vi "Teleop.vi"(10 "Match Info":T1={"Autonomous Elapsed Seconds"=0.0, "TeleOp Elapsed Seconds"=0.0, "Disabled Elapsed Seconds"=0.0, "Visited Autonomous"=FALSE, "Visited TeleOp"=FALSE, "Visited Disabled"=FALSE, "Autonomous Settings"={"Autonomous Style"=enum."Independent", "VI Refnum"=refnum}}, 11 "Call Context":T2) -> ()   [LabVIEW 2017]
doc: "This VI is called for each enabled TeleOp packet received from the DS. It is typically used to read from joysticks and other inputs and update I/O or setpoints for timed control loops. It should complete and return within 20 milliseconds or risk missing DS packets."
uses:
  <vilib>/Rock Robotics/WPI/DriverStation/WPI_DriverStationDerivedRobotMode.ctl
  <vilib>/Rock Robotics/WPI/DriverStation/WPI_DriverStationMatch Info.ctl
  <vilib>/Rock Robotics/WPI/Utilities/WPI_GetSetVariantRefNum.vi
  <vilib>/Rock Robotics/Network Tables/NT Write Boolean Array.vi
  <vilib>/Rock Robotics/Network Tables/NT Write Numeric Array.vi
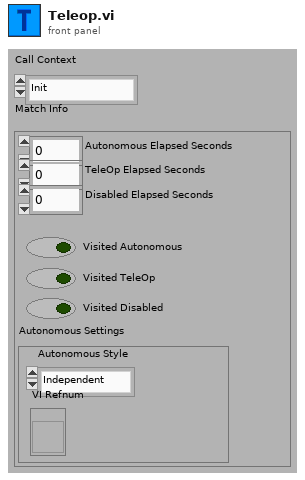
[diagram p1: front panel]
types:
  T1 = typedef "WPI_DriverStationMatch Info.ctl" = cluster{"Autonomous Elapsed Seconds":dbl, "TeleOp Elapsed Seconds":dbl, "Disabled Elapsed Seconds":dbl, "Visited Autonomous":bool, "Visited TeleOp":bool, "Visited Disabled":bool, "Autonomous Settings":cluster{"Autonomous Style":enum16{"Iterative", "Independent"}, "VI Refnum":refnum<vi>}}
  T2 = typedef "WPI_DriverStationDerivedRobotMode.ctl" = enum16{"Init", "Execute", "Stop"}
  T3 = typedef "WPI_JoystickDevRef.ctl" = cluster{"Device":T4}
  T4 = typedef "WPI_JoystickDeviceEnum.ctl" = enum16{"USB 0", "USB 1", "USB 2", "USB 3", "USB 4", "USB 5"}
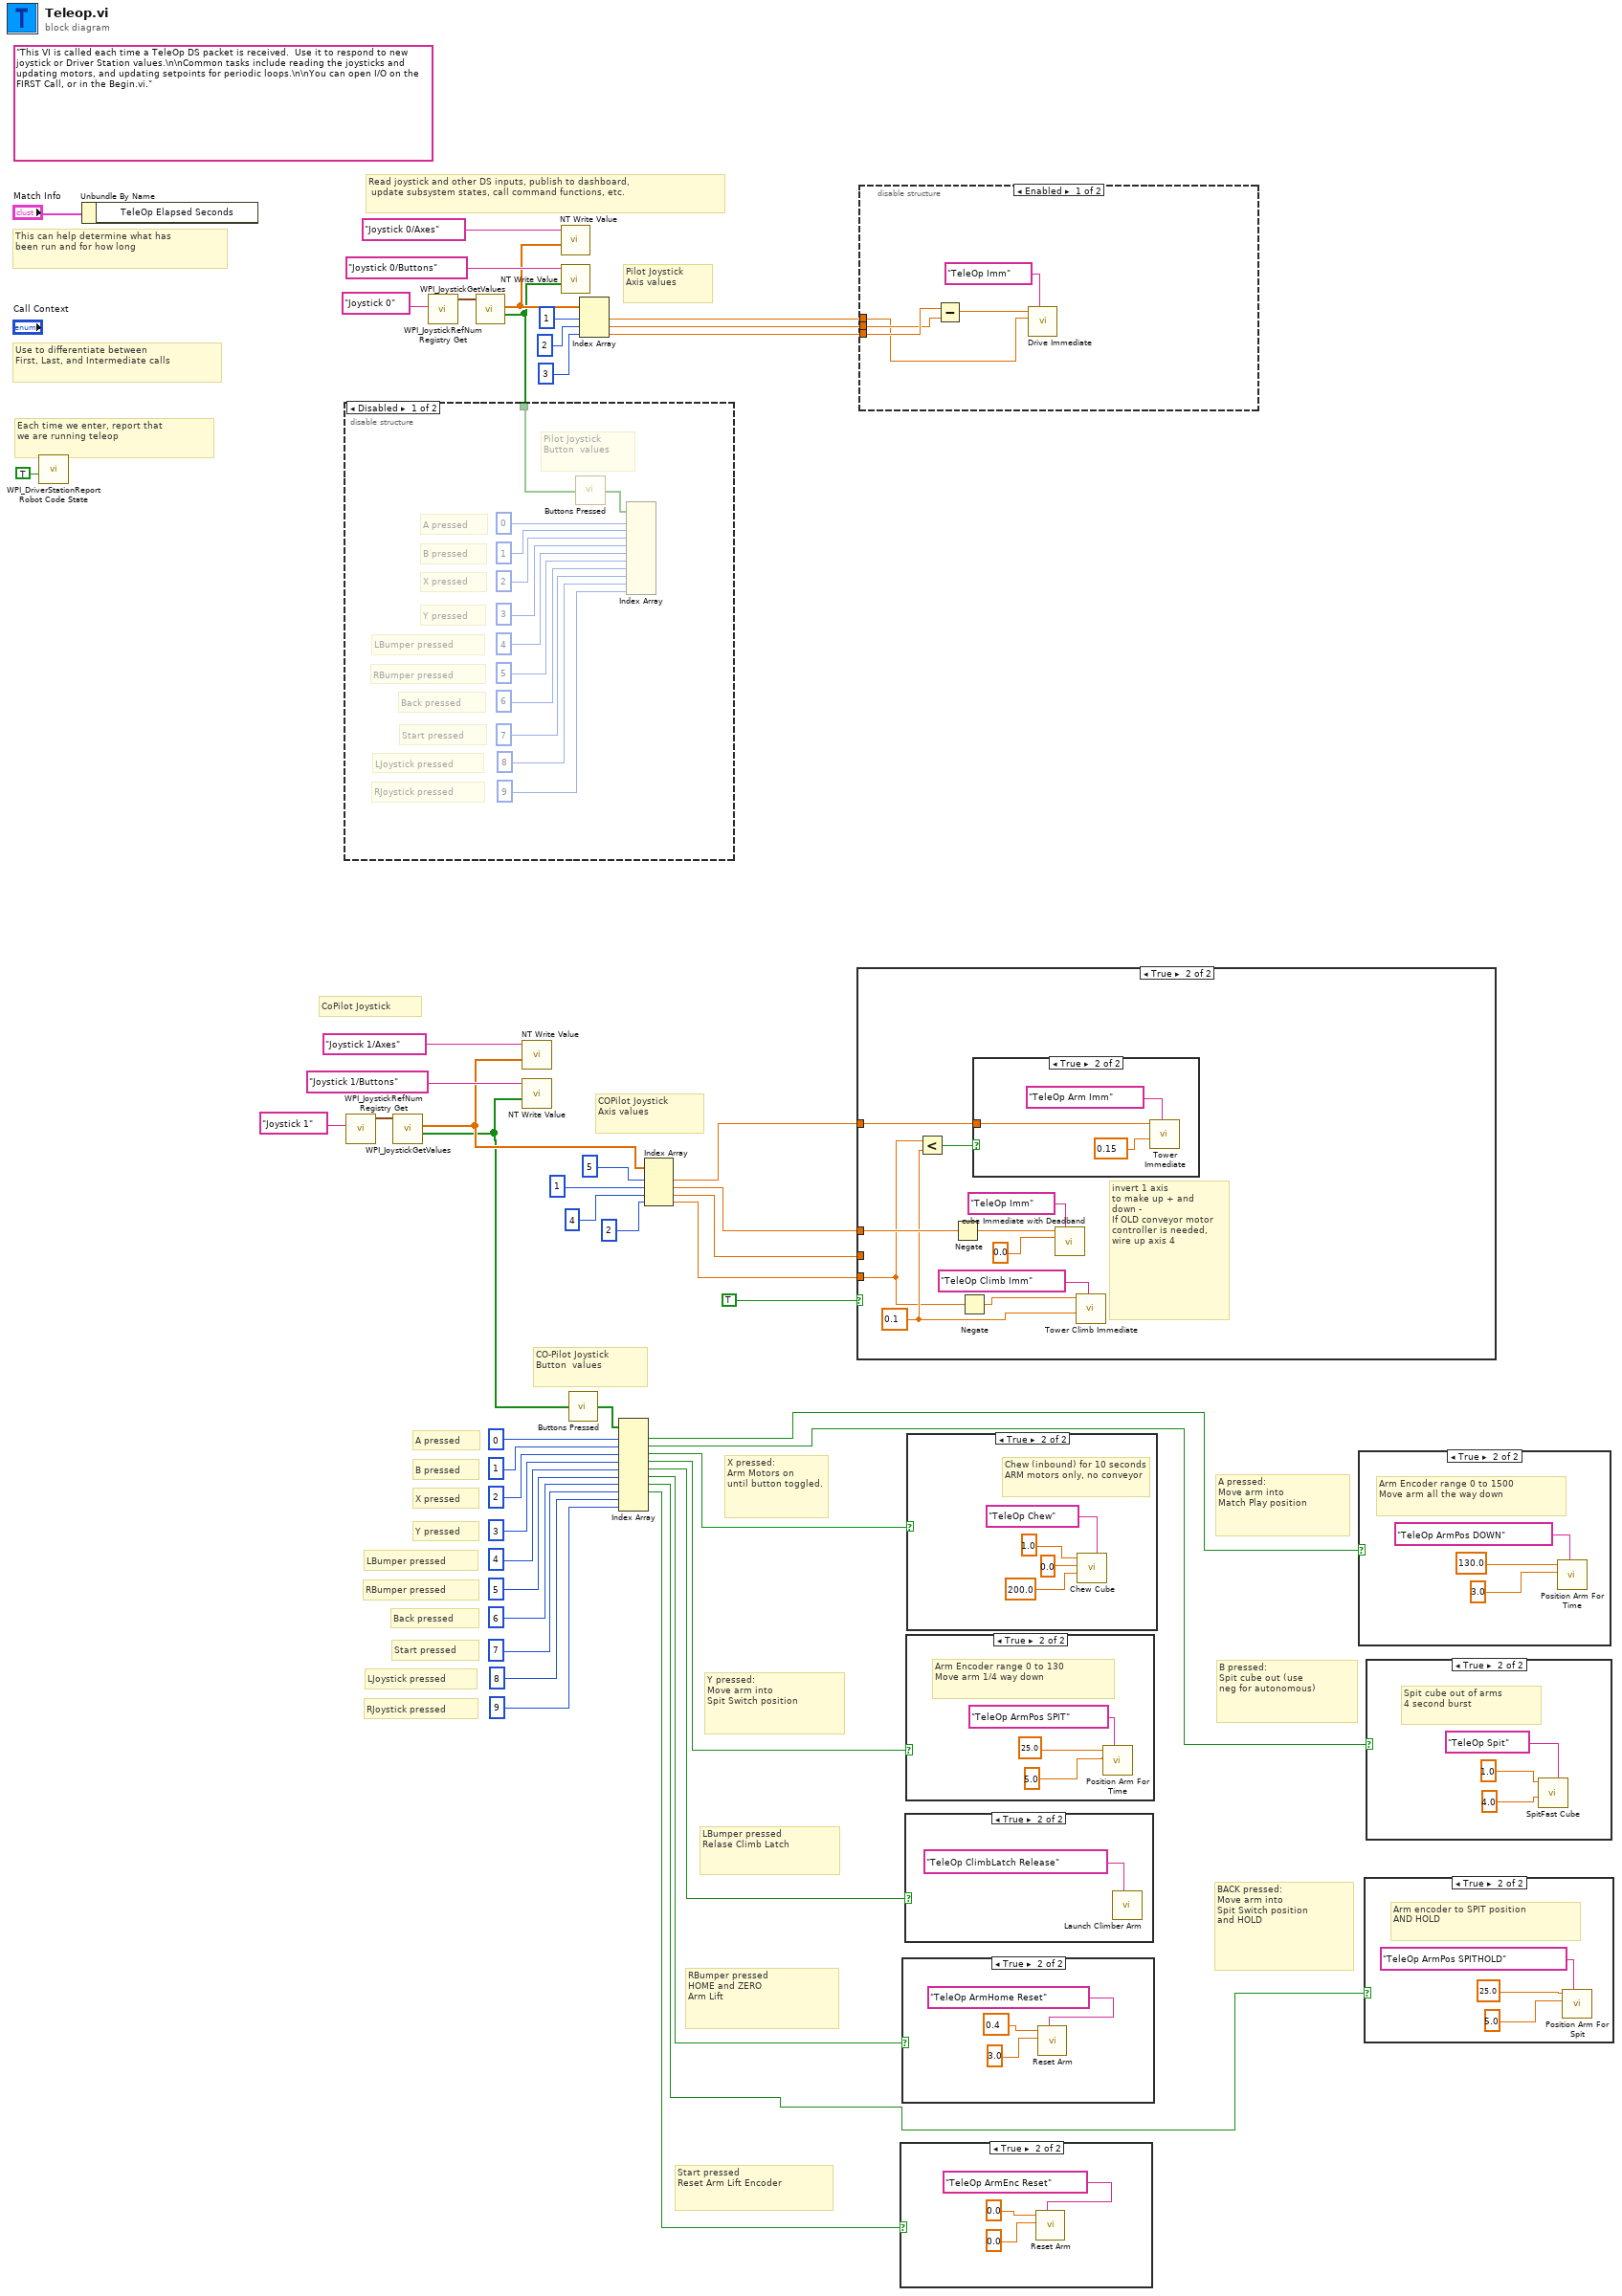
[diagram p0: block diagram]
diagram:
  (unwired) "This VI is called each time a TeleOp DS packet is received.  Use it to respond to new joystick or Driver Station values.\n\nCommon tasks include reading the joysticks and updating motors, and updating setpoints for periodic loops.\n\nYou can open I/O on the FIRST Call, or in the Begin.vi."
  # "BACK pressed:\nMove arm into\nSpit Switch position\nand HOLD"
  # "B pressed:\nSpit cube out (use\nneg for autonomous)"
  # "X pressed:\nArm Motors on\nuntil button toggled."
  # "Y pressed:\nMove arm into\nSpit Switch position"
  # "A pressed:\nMove arm into\nMatch Play position"
  # "LBumper pressed\nRelase Climb Latch"
  # "Start pressed\nReset Arm Lift Encoder"
  # "RBumper pressed\nHOME and ZERO\nArm Lift"
  # "LJoystick pressed"
  # "RJoystick pressed"
  # "LBumper pressed"
  # "Start pressed"
  # "Back pressed"
  # "RBumper pressed"
  # "A pressed"
  # "CO-Pilot Joystick \nButton  values"
  # "Y pressed"
  # "X pressed"
  # "B pressed"
  # "COPilot Joystick \nAxis values"
  # "Pilot Joystick \nAxis values"
  # "CoPilot Joystick"
  # "Read joystick and other DS inputs, publish to dashboard,\n update subsystem states, call command functions, etc."
  # "Each time we enter, report that\nwe are running teleop"
  # "Use to differentiate between\nFirst, Last, and Intermediate calls"
  # "This can help determine what has\nbeen run and for how long"
  n1 = call <vilib>:"WPI_DriverStationReport Robot Code State.vi"("TeleOp"=TRUE ("Autonomous")) -> ()  [unwired: 10 in, 1 out]
  n2 = Unbundle By Name("Match Info") -> ()  [unwired: 1 out]
  n3 = call <vilib>:"WPI_JoystickRefNum Registry Get.vi"("refnum name"="Joystick 1") -> ("JoystickDevRef"=w34:T3)  [unwired: 1 in, 9 out]
  n4 = call <vilib>:"WPI_JoystickGetValues.vi"("JoystickDevRef"=w34) -> ("Buttons"=w9:bool[], "Axes"=w31:dbl[])  [unwired: 6 in, 3 out]
  n5 = call <vilib>:"WPI_JoystickRefNum Registry Get.vi"("refnum name"="Joystick 0") -> ("JoystickDevRef"=w45:T3)  [unwired: 1 in, 9 out]
  n6 = call <vilib>:"WPI_JoystickGetValues.vi"("JoystickDevRef"=w45) -> ("Buttons"=w22:bool[], "Axes"=w43:dbl[])  [unwired: 6 in, 3 out]
  n7 = disable-structure shown="Disabled" {
    disable-tunnel: w22 -> [w59 _]
    frame Disabled {
      # "LJoystick pressed"
      # "RJoystick pressed"
      # "LBumper pressed"
      # "Start pressed"
      # "Back pressed"
      # "RBumper pressed"
      # "A pressed"
      # "Pilot Joystick \nButton  values"
      # "Y pressed"
      # "X pressed"
      # "B pressed"
      n8 = call "Buttons Pressed.vi"("Button Values"=w59) -> ("Button Presses"=w60:bool[])
      n9 = Index Array(array=w60, index #1=0 ("index"), index #2=1 ("index"), index #3=2 ("index"), index #4=3 ("index"), index #5=4 ("index"), index #6=5 ("index"), index #7=6 ("index"), index #8=7 ("index"), index #9=8 ("index"), index #10=9 ("index")) -> ()  [unwired: 10 out]
    }
    frame Enabled {
    }
  }
  n10 = call-poly <vilib>:"NT Write Value.vi"("Numeric Array"=w31, "Name"="Joystick 1/Axes") -> ()  [unwired: 9 in, 1 out]
  n11 = call-poly <vilib>:"NT Write Value.vi"("Boolean Array"=w9, "Name"="Joystick 1/Buttons") -> ()  [unwired: 9 in, 1 out]
  n12 = call-poly <vilib>:"NT Write Value.vi"("Numeric Array"=w43, "Name"="Joystick 0/Axes") -> ()  [unwired: 9 in, 1 out]
  n13 = call-poly <vilib>:"NT Write Value.vi"("Boolean Array"=w22, "Name"="Joystick 0/Buttons") -> ()  [unwired: 9 in, 1 out]
  n14 = call "Buttons Pressed.vi"("Button Values"=w9) -> ("Button Presses"=w20:bool[])
  n15 = Index Array(array=w43, index #1=1 ("index"), index #2=2 ("index"), index #3=3 ("index")) -> (element #1=w38:dbl, element #2=w37:dbl, element #3=w36:dbl)
  n16 = Index Array(array=w20, index #1=0 ("index"), index #2=1 ("index"), index #3=2 ("index"), index #4=3 ("index"), index #5=4 ("index"), index #6=5 ("index"), index #7=6 ("index"), index #8=7 ("index"), index #9=8 ("index"), index #10=9 ("index")) -> (element #1=w2:bool, element #2=w3:bool, element #3=w4:bool, element #4=w5:bool, element #5=w6:bool, element #6=w8:bool, element #7=w1:bool, element #8=w7:bool)  [unwired: 2 out]
  n17 = Index Array(array=w31, index #1=5 ("index"), index #2=1 ("index"), index #3=4 ("index"), index #4=2 ("index")) -> (element #1=w25:dbl, element #2=w27:dbl, element #3=w26:dbl, element #4=w23:dbl)
  n18 = case shown="True" TRUE {
    tunnel: w27 -> [_ w68]
    tunnel: w26 -> [_ _]
    tunnel: w25 -> [_ w62]
    tunnel: w23 -> [_ w63]
    frame False {
    }
    frame True {
      w65 = 0.1 ("Deadband Value")
      # "invert 1 axis\nto make up + and\ndown -\nIf OLD conveyor motor controller is needed, wire up axis 4"
      n19 = Less?(x=w63, y=w65) -> (x < y?=w66:bool)
      n20 = Negate(x=w68) -> (-x=w69:dbl)
      n21 = Negate(x=w63) -> (-x=w64:dbl)
      n22 = case shown="True" w66 {
        tunnel: w62 -> [_ w72]
        frame False {
        }
        frame True {
          n23 = call "Tower Immediate.vi"("Description"="TeleOp Arm Imm", "Deadband Value"=0.15, "Setpoint"=w72) -> ()  [unwired: 8 in, 1 out]
        }
      }
      n24 = call "cube Immediate with Deadband.vi"("Description"="TeleOp Imm", "Conveyor Setpoint"=0.0, "Arm Setpoint"=w69) -> ()  [unwired: 8 in, 1 out]
      n25 = call "Tower Climb Immediate.vi"("Description"="TeleOp Climb Imm", "Deadband Value"=w65, "Setpoint"=w64) -> ()  [unwired: 8 in, 1 out]
    }
  }
  n26 = disable-structure shown="Enabled" {
    disable-tunnel: w36 -> [w76 _]
    disable-tunnel: w37 -> [w75 _]
    disable-tunnel: w38 -> [w74 _]
    frame Enabled {
      n27 = Subtract(x=w76, y=w75) -> (x-y=w77:dbl)
      n28 = call "Drive Immediate.vi"("Description"="TeleOp Imm", "Right Setpoint"=w74, "Left Setpoint"=w77) -> ()  [unwired: 8 in, 1 out]
    }
    frame Disabled {
    }
  }
  n29 = case shown="True" w7 {
    frame False {
    }
    frame True {
      n30 = call "Reset Arm.vi"("Description"="TeleOp ArmEnc Reset", "Duration (secs)"=0.0, "Setpoint"=0.0) -> ()  [unwired: 8 in, 1 out]
    }
  }
  n31 = case shown="True" w8 {
    frame False {
    }
    frame True {
      n32 = call "Reset Arm.vi"("Description"="TeleOp ArmHome Reset", "Duration (secs)"=3.0, "Setpoint"=0.4) -> ()  [unwired: 8 in, 1 out]
    }
  }
  n33 = case shown="True" w6 {
    frame False {
    }
    frame True {
      n34 = call "Launch Climber Arm.vi"("Description"="TeleOp ClimbLatch Release") -> ()  [unwired: 10 in, 1 out]
    }
  }
  n35 = case shown="True" w5 {
    frame False {
    }
    frame True {
      # "Arm Encoder range 0 to 130\nMove arm 1/4 way down"
      n36 = call "Position Arm For Time.vi"("Description"="TeleOp ArmPos SPIT", "Duration (s)"=5.0, "Setpoint"=25.0) -> ()  [unwired: 8 in, 1 out]
    }
  }
  n37 = case shown="True" w4 {
    frame False {
    }
    frame True {
      # "Chew (inbound) for 10 seconds\nARM motors only, no conveyor"
      n38 = call "Chew Cube.vi"("Arm Setpoint"=1.0, "Conveyor Setpoint"=0.0 ("Arm Setpoint"), "Duration (s)"=200.0, "Description"="TeleOp Chew") -> ()  [unwired: 6 in, 1 out]
    }
  }
  n39 = case shown="True" w2 {
    frame False {
    }
    frame True {
      # "Arm Encoder range 0 to 1500\nMove arm all the way down"
      n40 = call "Position Arm For Time.vi"("Description"="TeleOp ArmPos DOWN", "Duration (s)"=3.0, "Setpoint"=130.0) -> ()  [unwired: 8 in, 1 out]
    }
  }
  n41 = case shown="True" w1 {
    frame False {
    }
    frame True {
      # "Arm encoder to SPIT position\nAND HOLD"
      n42 = call "Position Arm For Spit.vi"("Description"="TeleOp ArmPos SPITHOLD", "Duration (s)"=5.0, "Setpoint"=25.0) -> ()  [unwired: 8 in, 1 out]
    }
  }
  n43 = case shown="True" w3 {
    frame False {
    }
    frame True {
      # "Spit cube out of arms\n4 second burst"
      n44 = call "SpitFast Cube.vi"("Arm Setpoint"=1.0, "Duration (s)"=4.0, "Description"="TeleOp Spit") -> ()  [unwired: 7 in, 1 out]
    }
  }
